vi "Create.vi"(8 "error in (no error)":errorcluster) -> (0 "error out":errorcluster, 3 "Dictionary out":refnum<class "Dictionary.lvclass">)   [LabVIEW 2018, in "Application.lvlib" / "Dictionary.lvclass"]
uses:
  Dictionary.lvclass
  Dictionary.lvclass/Dictionary.ctl
panel:
  in  "Dictionary in":refnum<class "Dictionary.lvclass">
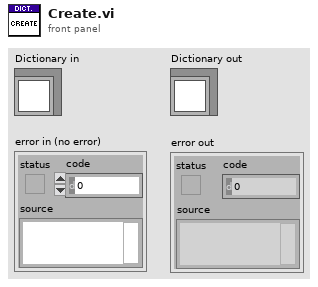
[diagram p1: front panel]
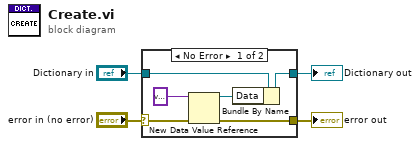
[diagram p0: block diagram]
diagram:
  n1 = case shown="No Error" "error in (no error)" {
    selector: "error in (no error)" -> [w10 w12]
    tunnel: [w5 w12] -> w3
    tunnel: [w6 w11] -> w1
    tunnel: "Dictionary in" -> [w7 w11]
    frame No Error {
      n2 = New Data Value Reference(data value=variant, error in=w10) -> (data value reference=w8:refnum<data-value>, error out=w5:errorcluster)
      n3 = Bundle By Name(cluster=w7, "Data"=w8) -> (w6:refnum<class "Dictionary.lvclass">)
    }
    frame Error {
    }
  }
  "error out" <- w3
  "Dictionary out" <- w1
